vi "FLUKE_8845A.vi"() -> ()   [LabVIEW 2020]
uses:
  <vilib>/Instr/_visa.llb/VISA Configure Serial Port (Instr).vi
  <vilib>/Utility/file.llb/Write Delimited Spreadsheet (DBL).vi
panel:
  in  "Device 2":refnum<visa-resource-name>="COM4"
  in  "Function 2":u16(ring) caption="Function" items=["AC Current", "DC Current", "AC Voltage", "DC Voltage", "Resistance"]
  in  "Clear 2":bool
  in  "Save Stop 2":bool caption="Save Stop"
  in  "Save Start 2":bool caption="Save Start"
  out "Save Time 2":timestamp
  out "Save Data 2":dbl[](array[numeric]) caption="Save Data"
  out "Device2 Buffer":string
  out "Preview graph 2":cluster{dbl[], "array":dbl[]}(graph)
  out "Saving 2":bool caption="Saving"
  out "read buffer 2":string caption="Read Buffer"
  out "Change 2":bool caption="Change"
  in  "Save Path 2":path caption="Save Path"
  out "=> 2":bool
  out "OVERLOAD 2":bool caption="OVERLOAD"
  out "Preview graph":cluster{dbl[], "array":dbl[]}(graph)
  out "Save Time":timestamp
  in  "stop":bool
  out "OVERLOAD":bool
  out "=>":bool
  out "Device1 Buffer":string
  in  "Save Path":path
  in  "Clear":bool
  out "Change":bool
  out "Save Data":dbl[](array[numeric])
  out "Saving":bool
  in  "Save Stop":bool
  in  "Save Start":bool
  in  "Function":u16(ring) items=["AC Current", "DC Current", "AC Voltage", "DC Voltage", "Resistance"]
  out "read buffer":string caption="Read Buffer"
  in  "Device 1":refnum<visa-resource-name>="COM4"
  # "made by Ji Won Kim  2021.06.17"
  # "Digit Precision Multimeter Controller"
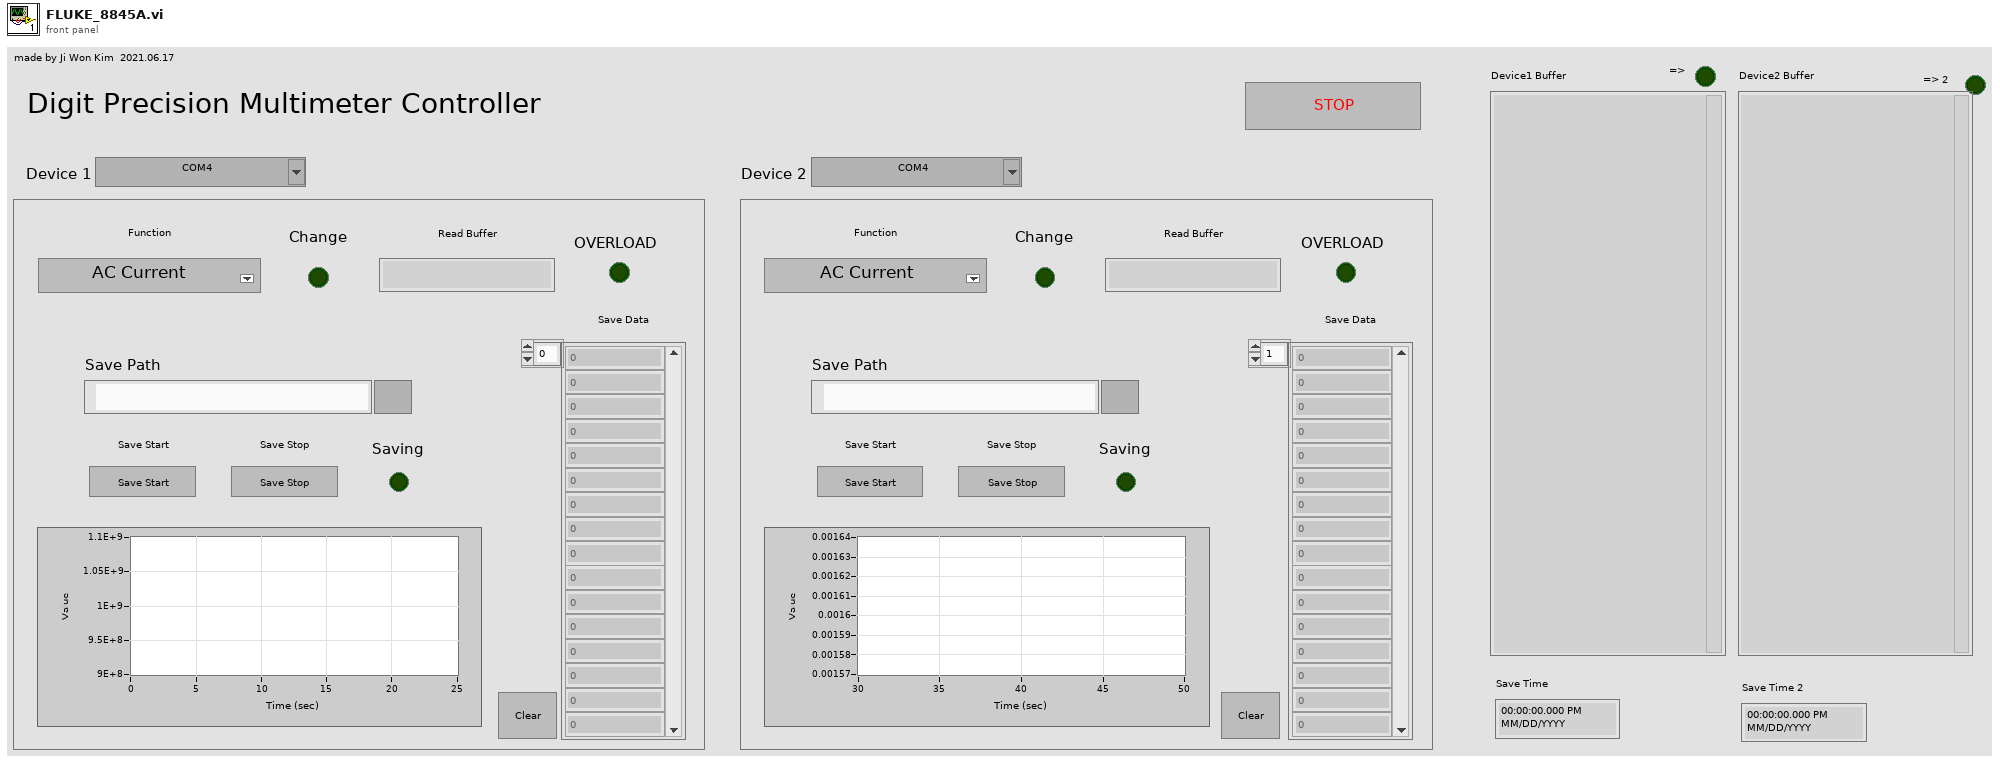
[diagram p1: front panel]
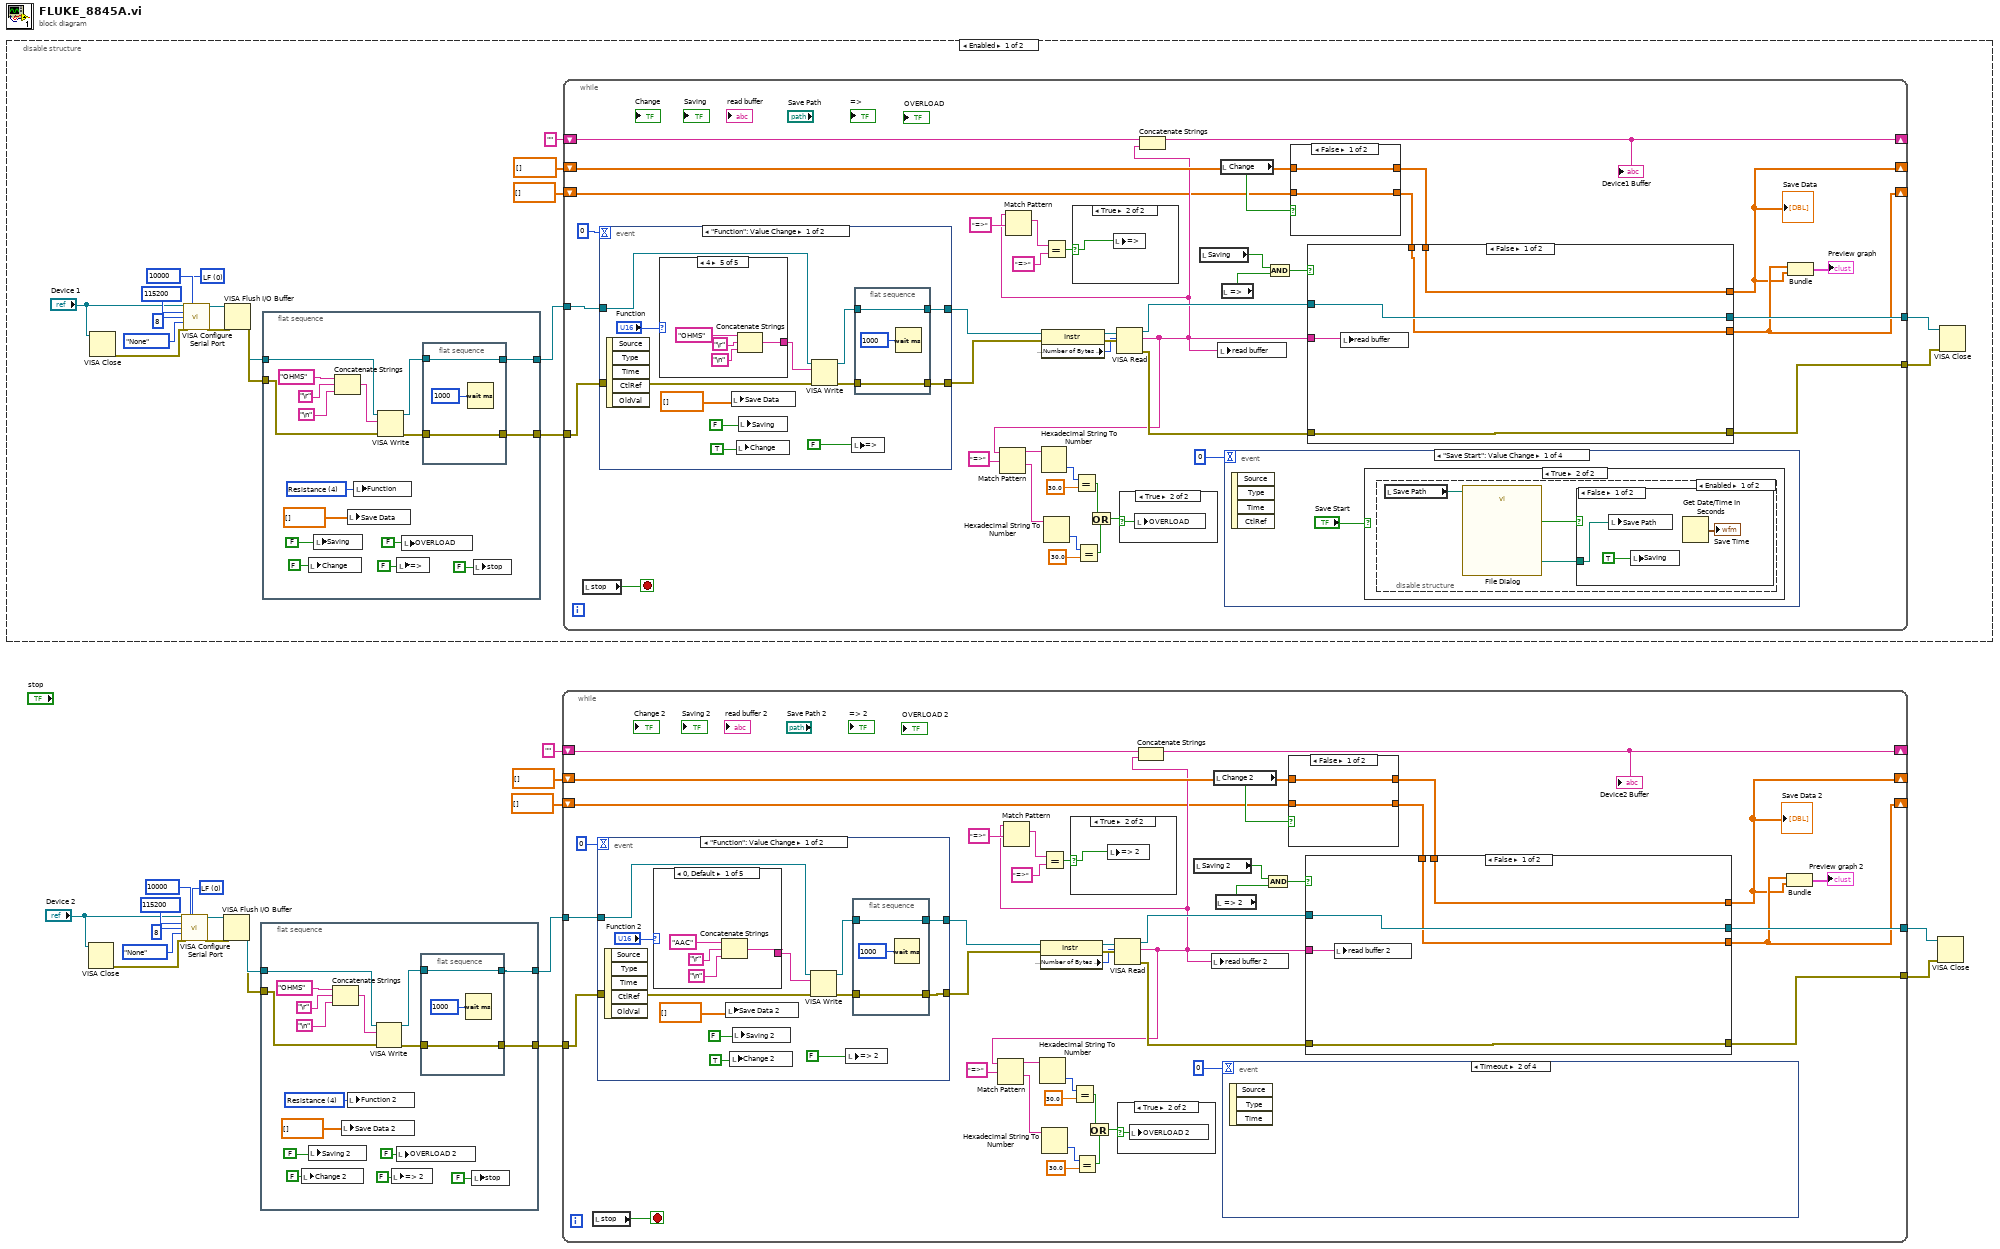
[diagram p0: block diagram]
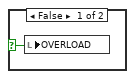
[diagram p2: hidden frame]
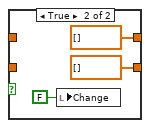
[diagram p4: hidden frame]
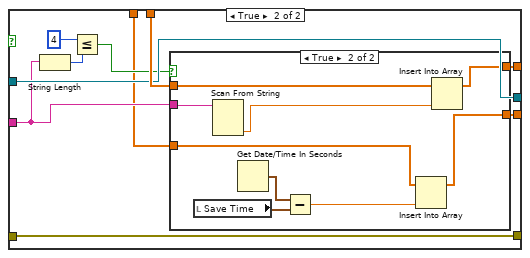
[diagram p5: hidden frame]
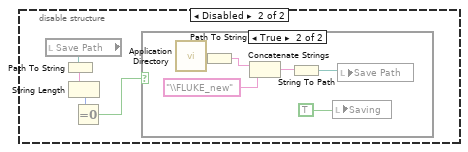
[diagram p9: hidden frame]
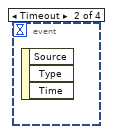
[diagram p11: hidden frame]
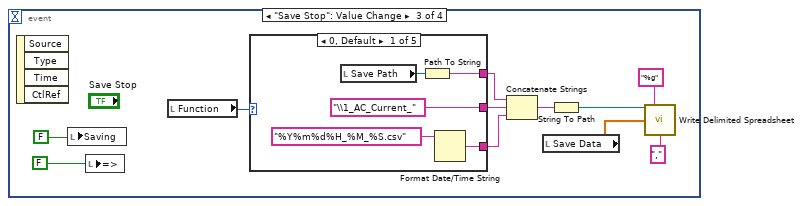
[diagram p12: hidden frame]
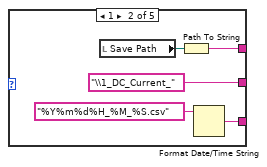
[diagram p13: hidden frame]
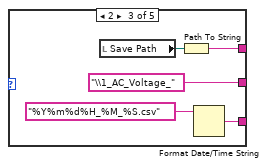
[diagram p14: hidden frame]
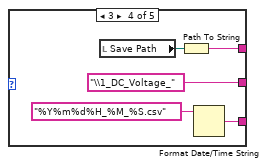
[diagram p15: hidden frame]
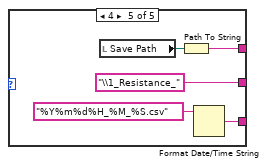
[diagram p16: hidden frame]
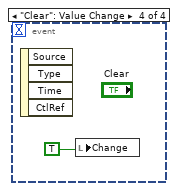
[diagram p17: hidden frame]
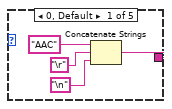
[diagram p18: hidden frame]
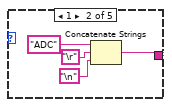
[diagram p19: hidden frame]
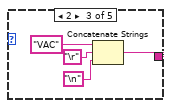
[diagram p20: hidden frame]
diagram:
  w3 = u16 0 items=["LF"]
  n1 = disable-structure shown="Enabled" {
    frame Enabled {
      w35 = u16 0 items=["LF"]
      n2 = VISA Close(VISA resource name="Device 1") -> (error out=w31:errorcluster)  [unwired: 1 in]
      n3 = call-poly "VISA Configure Serial Port"("VISA resource name"="Device 1", "timeout (10sec)"=u32 10000, "termination char\n(0xA = '\\n' = LF)"=w35, "baud rate (9600)"=u32 115200, "data bits (8)"=u16 8, "parity (0:none)"=enum16{"None", "Odd", "Even", "Mark", "Space"}."None", "error in (no error)"=w31) -> ("VISA resource name out"=w25:refnum<visa-resource-name>, "error out"=w24:errorcluster)  [unwired: 7 in]
      n4 = VISA Flush I/O Buffer(VISA resource name=w25, error in (no error)=w24) -> (VISA resource name out=w22:refnum<visa-resource-name>, error out=w23:errorcluster)  [unwired: 1 in]
      n5 = flat-sequence {
        tunnel: w22 -> [w46]
        tunnel: w23 -> [w45]
        tunnel: [w44] -> w27
        tunnel: [w43] -> w26
        frame #0 {
          w53 = u16 4 items=["AC Current", "DC Current", "AC Voltage", "DC Voltage", "Resistance"] ("Function")
          n6 = local write "Change"(FALSE ("Change")) -> ()
          n7 = local write "Saving"(FALSE ("Saving")) -> ()
          n8 = Concatenate Strings("OHMS" ("string"), "\r", "\n") -> (w52:string)
          n9 = local write "Save Data"(dbl[] [] ("array")) -> ()
          n10 = local write "Function"(w53) -> ()
          n11 = VISA Write(VISA resource name=w46, write buffer=w52, error in (no error)=w45) -> (VISA resource name out=w50:refnum<visa-resource-name>, error out=w51:errorcluster)  [unwired: 1 out]
          n12 = local write "=>"(FALSE ("Value Change")) -> ()
          n13 = local write "OVERLOAD"(FALSE ("OVERLOAD")) -> ()
          n14 = flat-sequence {
            tunnel: [w55] -> w44
            tunnel: w50 -> [w55]
            tunnel: [w54] -> w43
            tunnel: w51 -> [w54]
            frame #0 {
              n15 = Wait (ms)(milliseconds to wait=u32 1000) -> ()  [unwired: 1 out]
            }
          }
          n16 = local write "stop"(FALSE ("stop")) -> ()
        }
      }
      n17 = while {
        tunnel: [w88] -> w29
        tunnel: [w90] -> w28
        tunnel: w27 -> [w92]
        tunnel: w26 -> [w91]
        shift-right: [w57] -> _
        shift-left: dbl[] [] -> [w84]
        shift-right: [w82] -> _
        shift-left: "" -> [w81]
        shift-right: [w58] -> _
        shift-left: dbl[] [] ("array") -> [w60]
        stop <- w62 stop-if-true
        n18 = local read "stop"() -> (w62:bool)
        n19 = event shown="[0] \"Function\": Value Change" {
          selector: _ -> [_ _]
          dyn-events: _ -> [_ _]
          timeout: 0 -> [_ _]
          tunnel: [w196 w225] -> w95
          tunnel: [w194 w224] -> w94
          tunnel: w92 -> [w192 w223]
          tunnel: w91 -> [w191 w222]
          event "Function": Value Change {
            n20 = event-data() -> ()  [unwired: 1 in, 5 out]
            n21 = case shown="4" "Function" {
              tunnel: [w204 w208 w212 w216 w220] -> w197
              frame 0, Default {
                n22 = Concatenate Strings("AAC" ("string"), "\r", "\n") -> (w204:string)
              }
              frame 1 {
                n23 = Concatenate Strings("ADC" ("string"), "\r", "\n") -> (w208:string)
              }
              frame 2 {
                n24 = Concatenate Strings("VAC" ("string"), "\r", "\n") -> (w212:string)
              }
              frame 3 {
                n25 = Concatenate Strings("VDC" ("string"), "\r", "\n") -> (w216:string)
              }
              frame 4 {
                n26 = Concatenate Strings("OHMS" ("string"), "\r", "\n") -> (w220:string)
              }
            }
            n27 = local write "Save Data"(dbl[] [] ("array")) -> ()
            n28 = local write "Change"(TRUE ("Change")) -> ()
            n29 = local write "Saving"(FALSE ("Saving")) -> ()
            n30 = VISA Write(VISA resource name=w192, write buffer=w197, error in (no error)=w191) -> (VISA resource name out=w195:refnum<visa-resource-name>, error out=w193:errorcluster)  [unwired: 1 out]
            n31 = local write "=>"(FALSE ("Value Change")) -> ()
            n32 = flat-sequence {
              tunnel: [w199] -> w196
              tunnel: w195 -> [w199]
              tunnel: [w200] -> w194
              tunnel: w193 -> [w200]
              frame #0 {
                n33 = Wait (ms)(milliseconds to wait=u32 1000) -> ()  [unwired: 1 out]
              }
            }
          }
          event Timeout {
            n34 = event-data() -> ()  [unwired: 1 in, 3 out]
            n35 = Concatenate Strings("MEAS1?" ("string"), "\r", "\n") -> (w231:string)
            n36 = VISA Write(VISA resource name=w223, write buffer=w231, error in (no error)=w222) -> (VISA resource name out=w230:refnum<visa-resource-name>, error out=w229:errorcluster)  [unwired: 1 out]
            n37 = flat-sequence {
              tunnel: [w233] -> w225
              tunnel: w230 -> [w233]
              tunnel: [w232] -> w224
              tunnel: w229 -> [w232]
              frame #0 {
                n38 = Wait (ms)(milliseconds to wait=u32 1000) -> ()  [unwired: 1 out]
              }
            }
          }
        }
        n39 = property class="Instr"(reference=w95, error in=w94) -> (reference out=w98:refnum<visa-resource-name>, error out=w97:errorcluster, "Serial Settings:Number of Bytes at Serial Port"=w96:u32)
        n40 = VISA Read(VISA resource name=w98, byte count=w96, error in (no error)=w97) -> (VISA resource name out=w89:refnum<visa-resource-name>, read buffer=w73:string, error out=w87:errorcluster)  [unwired: 1 out]
        n41 = Match Pattern(string=w73, regular expression="=>" ("x")) -> (before substring=w69:string, after substring=w66:string)  [unwired: 1 in, 2 out]
        n42 = Match Pattern(string=w73, regular expression="=>" ("x")) -> (match substring=w77:string)  [unwired: 1 in, 3 out]
        n43 = Hexadecimal String To Number(string=w69) -> (number=w70:u32)  [unwired: 2 in, 1 out]
        n44 = Equal?(x=w77, y="=>" ("x")) -> (x = y?=w75:bool)
        n45 = Hexadecimal String To Number(string=w66) -> (number=w68:u32)  [unwired: 2 in, 1 out]
        n46 = case shown="True" w75 {
          selector: w75 -> [_ w101]
          frame False {
          }
          frame True {
            n47 = local write "=>"(w101) -> ()
          }
        }
        n48 = Equal?(x=w70, y=30.0) -> (x = y?=w65:bool)
        n49 = Equal?(x=w68, y=30.0) -> (x = y?=w64:bool)
        n50 = Or(x=w65, y=w64) -> (x .or. y?=w63:bool)
        n51 = case shown="True" w63 {
          selector: w63 -> [w99 w100]
          frame False {
            n52 = local write "OVERLOAD"(w99) -> ()
          }
          frame True {
            n53 = local write "OVERLOAD"(w100) -> ()
          }
        }
        n54 = Concatenate Strings(w81, w73) -> (w82:string)
        "Device1 Buffer" <- w82
        n55 = local read "Saving"() -> (w80:bool)
        n56 = local write "read buffer"(w73) -> ()
        n57 = local read "Change"() -> (w83:bool)
        n58 = local read "=>"() -> (w79:bool)
        n59 = event shown="[0] \"Save Start\": Value Change" {
          selector: _ -> [_ _ _ _]
          dyn-events: _ -> [_ _ _ _]
          timeout: 0 -> [_ _ _ _]
          event "Save Start": Value Change {
            n60 = event-data() -> ()  [unwired: 1 in, 4 out]
            n61 = case shown="True" "Save Start" {
              frame False {
              }
              frame True {
                n62 = disable-structure shown="Enabled" {
                  frame Enabled {
                    n63 = local read "Save Path"() -> (w134:path)
                    n64 = call "File Dialog"("start path"=w134) -> ("selected path"=w136:path, "cancelled"=w135:bool)  [unwired: 11 in, 2 out]
                    n65 = case shown="False" w135 {
                      tunnel: w136 -> [w138 _]
                      frame False {
                        n66 = local write "Save Path"(w138) -> ()
                        n67 = local write "Saving"(TRUE ("Saving")) -> ()
                        n68 = Get Date/Time In Seconds() -> (seconds since 1Jan1904=→"Save Time":timestamp)
                      }
                      frame True {
                      }
                    }
                  }
                  frame Disabled {
                    n69 = local read "Save Path"() -> (w143:path)
                    n70 = Path To String(path=w143) -> (string=w142:string)
                    n71 = String Length(string=w142) -> (length=w141:i32)
                    n72 = Equal To 0?(x=w141) -> (x = 0?=w140:bool)
                    n73 = case shown="True" w140 {
                      frame False {
                      }
                      frame True {
                        n74 = call <vilib>:"Application Directory.vi"() -> ("Application Directory"=w149:path)
                        n75 = Path To String(path=w149) -> (string=w148:string)
                        n76 = Concatenate Strings(w148, "\\FLUKE_new" ("string")) -> (w146:string)
                        n77 = String To Path(string=w146) -> (path=w145:path)
                        n78 = local write "Saving"(TRUE ("Saving")) -> ()
                        n79 = local write "Save Path"(w145) -> ()
                      }
                    }
                  }
                }
              }
            }
          }
          event Timeout {
            n80 = event-data() -> ()  [unwired: 1 in, 3 out]
          }
          event "Save Stop": Value Change {
            n81 = event-data() -> ()  [unwired: 1 in, 4 out]
            n82 = local write "Saving"(FALSE ("Saving")) -> ()
            n83 = local write "=>"(FALSE ("Value Change")) -> ()
            n84 = local read "Function"() -> (w155:u16)
            n85 = case shown="0, Default" w155 {
              tunnel: [w163 w168 w173 w178 w183] -> w156
              tunnel: ["\\1_AC_Current_" ("time format string (%c)") "\\1_DC_Current_" ("time format string (%c)") "\\1_AC_Voltage_" ("time format string (%c)") "\\1_DC_Voltage_" ("time format string (%c)") "\\1_Resistance_" ("time format string (%c)")] -> w157
              tunnel: [w161 w166 w171 w176 w181] -> w158
              frame 0, Default {
                n86 = local read "Save Path"() -> (w164:path)
                n87 = Path To String(path=w164) -> (string=w163:string)
                n88 = Format Date/Time String(time format string (%c)="%Y%m%d%H_%M_%S.csv") -> (date/time string=w161:string)  [unwired: 2 in]
              }
              frame 1 {
                n89 = local read "Save Path"() -> (w169:path)
                n90 = Path To String(path=w169) -> (string=w168:string)
                n91 = Format Date/Time String(time format string (%c)="%Y%m%d%H_%M_%S.csv") -> (date/time string=w166:string)  [unwired: 2 in]
              }
              frame 2 {
                n92 = local read "Save Path"() -> (w174:path)
                n93 = Path To String(path=w174) -> (string=w173:string)
                n94 = Format Date/Time String(time format string (%c)="%Y%m%d%H_%M_%S.csv") -> (date/time string=w171:string)  [unwired: 2 in]
              }
              frame 3 {
                n95 = local read "Save Path"() -> (w179:path)
                n96 = Path To String(path=w179) -> (string=w178:string)
                n97 = Format Date/Time String(time format string (%c)="%Y%m%d%H_%M_%S.csv") -> (date/time string=w176:string)  [unwired: 2 in]
              }
              frame 4 {
                n98 = local read "Save Path"() -> (w184:path)
                n99 = Path To String(path=w184) -> (string=w183:string)
                n100 = Format Date/Time String(time format string (%c)="%Y%m%d%H_%M_%S.csv") -> (date/time string=w181:string)  [unwired: 2 in]
              }
            }
            n101 = Concatenate Strings(w156, w157, w158) -> (w154:string)
            n102 = local read "Save Data"() -> (w151:dbl[])
            n103 = String To Path(string=w154) -> (path=w159:path)
            n104 = call-poly <vilib>:"Write Delimited Spreadsheet.vi"("file path (dialog if empty)"=w159, "format (%.3f)"="%g", "1D data"=w151, "delimiter (\\t)"="," ("delimiter (\\t)")) -> ()  [unwired: 10 in, 2 out]
          }
          event "Clear": Value Change {
            n105 = event-data() -> ()  [unwired: 1 in, 4 out]
            n106 = local write "Change"(TRUE ("Change")) -> ()
          }
        }
        n107 = And(x=w80, y=w79) -> (x .and. y?=w74:bool)
        n108 = case shown="False" w83 {
          tunnel: [w103 dbl[] []] -> w85
          tunnel: w84 -> [w103 _]
          tunnel: [w102 dbl[] [] ("array")] -> w61
          tunnel: w60 -> [w102 _]
          frame False {
          }
          frame True {
            n109 = local write "Change"(FALSE ("Change")) -> ()
          }
        }
        n110 = case shown="False" w74 {
          tunnel: w85 -> [w109 w121]
          tunnel: [w111 w120] -> w90
          tunnel: w89 -> [w111 w120]
          tunnel: [w110 w119] -> w88
          tunnel: w87 -> [w110 w119]
          tunnel: [w109 w118] -> w57
          tunnel: w73 -> [w108 w114]
          tunnel: w61 -> [w107 w113]
          tunnel: [w107 w112] -> w58
          frame False {
            n111 = local write "read buffer"(w108) -> ()
          }
          frame True {
            n112 = String Length(string=w114) -> (length=w117:i32)
            n113 = Less Or Equal?(x=4, y=w117) -> (x <= y?=w115:bool)
            n114 = case shown="True" w115 {
              tunnel: w121 -> [w123 w128]
              tunnel: [w123 w129] -> w118
              tunnel: w114 -> [_ w132]
              tunnel: w113 -> [w122 w125]
              tunnel: [w122 w124] -> w112
              frame False {
              }
              frame True {
                n115 = local read "Save Time"() -> (w130:timestamp)
                n116 = Scan From String(input string=w132) -> (output 1=w127:dbl)  [unwired: 4 in, 3 out]
                n117 = Get Date/Time In Seconds() -> (seconds since 1Jan1904=w131:timestamp)
                n118 = Subtract(x=w131, y=w130) -> (x-y=w126:dbl)
                n119 = Insert Into Array(array=w125, new element=w126) -> (w124:dbl[])  [unwired: 1 in]
                n120 = Insert Into Array(array=w128, new element=w127) -> (w129:dbl[])  [unwired: 1 in]
              }
            }
          }
        }
        "Save Data" <- w57
        n121 = Bundle("array"=w58, w57) -> (→"Preview graph":cluster{"array":dbl[], dbl[]})  [unwired: 1 in]
      }
      n122 = VISA Close(VISA resource name=w28, error in (no error)=w29) -> ()  [unwired: 1 out]
    }
    frame Disabled {
    }
  }
  n123 = VISA Close(VISA resource name="Device 2") -> (error out=w7:errorcluster)  [unwired: 1 in]
  n124 = call-poly "VISA Configure Serial Port"("VISA resource name"="Device 2", "timeout (10sec)"=u32 10000, "termination char\n(0xA = '\\n' = LF)"=w3, "baud rate (9600)"=u32 115200, "data bits (8)"=u16 8, "parity (0:none)"=enum16{"None", "Odd", "Even", "Mark", "Space"}."None", "error in (no error)"=w7) -> ("VISA resource name out"=w12:refnum<visa-resource-name>, "error out"=w13:errorcluster)  [unwired: 7 in]
  n125 = VISA Flush I/O Buffer(VISA resource name=w12, error in (no error)=w13) -> (VISA resource name out=w15:refnum<visa-resource-name>, error out=w14:errorcluster)  [unwired: 1 in]
  n126 = flat-sequence {
    tunnel: w15 -> [w244]
    tunnel: w14 -> [w243]
    tunnel: [w242] -> w10
    tunnel: [w241] -> w11
    frame #0 {
      w251 = u16 4 items=["AC Current", "DC Current", "AC Voltage", "DC Voltage", "Resistance"] ("Function")
      n127 = local write "Change 2"(FALSE ("Change")) -> ()
      n128 = local write "Saving 2"(FALSE ("Saving")) -> ()
      n129 = Concatenate Strings("OHMS" ("string"), "\r", "\n") -> (w250:string)
      n130 = local write "Save Data 2"(dbl[] [] ("array")) -> ()
      n131 = local write "Function 2"(w251) -> ()
      n132 = VISA Write(VISA resource name=w244, write buffer=w250, error in (no error)=w243) -> (VISA resource name out=w248:refnum<visa-resource-name>, error out=w249:errorcluster)  [unwired: 1 out]
      n133 = local write "=> 2"(FALSE ("Value Change")) -> ()
      n134 = local write "OVERLOAD 2"(FALSE ("OVERLOAD")) -> ()
      n135 = flat-sequence {
        tunnel: [w253] -> w242
        tunnel: w248 -> [w253]
        tunnel: [w252] -> w241
        tunnel: w249 -> [w252]
        frame #0 {
          n136 = Wait (ms)(milliseconds to wait=u32 1000) -> ()  [unwired: 1 out]
        }
      }
      n137 = local write "stop"(FALSE ("stop")) -> ()
    }
  }
  n138 = while {
    tunnel: [w286] -> w8
    tunnel: [w288] -> w9
    tunnel: w10 -> [w290]
    tunnel: w11 -> [w289]
    shift-right: [w255] -> _
    shift-left: dbl[] [] -> [w282]
    shift-right: [w280] -> _
    shift-left: "" -> [w279]
    shift-right: [w256] -> _
    shift-left: dbl[] [] ("array") -> [w258]
    stop <- w260 stop-if-true
    n139 = local read "stop"() -> (w260:bool)
    n140 = event shown="[0] \"Function\": Value Change" {
      selector: _ -> [_ _]
      dyn-events: _ -> [_ _]
      timeout: 0 -> [_ _]
      tunnel: [w394 w423] -> w293
      tunnel: [w392 w422] -> w292
      tunnel: w290 -> [w390 w421]
      tunnel: w289 -> [w389 w420]
      event "Function": Value Change {
        n141 = event-data() -> ()  [unwired: 1 in, 5 out]
        n142 = case shown="0, Default" "Function 2" {
          tunnel: [w402 w406 w410 w414 w418] -> w395
          frame 0, Default {
            n143 = Concatenate Strings("AAC" ("string"), "\r", "\n") -> (w402:string)
          }
          frame 1 {
            n144 = Concatenate Strings("ADC" ("string"), "\r", "\n") -> (w406:string)
          }
          frame 2 {
            n145 = Concatenate Strings("VAC" ("string"), "\r", "\n") -> (w410:string)
          }
          frame 3 {
            n146 = Concatenate Strings("VDC" ("string"), "\r", "\n") -> (w414:string)
          }
          frame 4 {
            n147 = Concatenate Strings("OHMS" ("string"), "\r", "\n") -> (w418:string)
          }
        }
        n148 = local write "Save Data 2"(dbl[] [] ("array")) -> ()
        n149 = local write "Change 2"(TRUE ("Change")) -> ()
        n150 = local write "Saving 2"(FALSE ("Saving")) -> ()
        n151 = VISA Write(VISA resource name=w390, write buffer=w395, error in (no error)=w389) -> (VISA resource name out=w393:refnum<visa-resource-name>, error out=w391:errorcluster)  [unwired: 1 out]
        n152 = local write "=> 2"(FALSE ("Value Change")) -> ()
        n153 = flat-sequence {
          tunnel: [w397] -> w394
          tunnel: w393 -> [w397]
          tunnel: [w398] -> w392
          tunnel: w391 -> [w398]
          frame #0 {
            n154 = Wait (ms)(milliseconds to wait=u32 1000) -> ()  [unwired: 1 out]
          }
        }
      }
      event Timeout {
        n155 = event-data() -> ()  [unwired: 1 in, 3 out]
        n156 = Concatenate Strings("MEAS1?" ("string"), "\r", "\n") -> (w429:string)
        n157 = VISA Write(VISA resource name=w421, write buffer=w429, error in (no error)=w420) -> (VISA resource name out=w428:refnum<visa-resource-name>, error out=w427:errorcluster)  [unwired: 1 out]
        n158 = flat-sequence {
          tunnel: [w431] -> w423
          tunnel: w428 -> [w431]
          tunnel: [w430] -> w422
          tunnel: w427 -> [w430]
          frame #0 {
            n159 = Wait (ms)(milliseconds to wait=u32 1000) -> ()  [unwired: 1 out]
          }
        }
      }
    }
    n160 = property class="Instr"(reference=w293, error in=w292) -> (reference out=w296:refnum<visa-resource-name>, error out=w295:errorcluster, "Serial Settings:Number of Bytes at Serial Port"=w294:u32)
    n161 = VISA Read(VISA resource name=w296, byte count=w294, error in (no error)=w295) -> (VISA resource name out=w287:refnum<visa-resource-name>, read buffer=w271:string, error out=w285:errorcluster)  [unwired: 1 out]
    n162 = Match Pattern(string=w271, regular expression="=>" ("x")) -> (before substring=w267:string, after substring=w264:string)  [unwired: 1 in, 2 out]
    n163 = Match Pattern(string=w271, regular expression="=>" ("x")) -> (match substring=w275:string)  [unwired: 1 in, 3 out]
    n164 = Hexadecimal String To Number(string=w267) -> (number=w268:u32)  [unwired: 2 in, 1 out]
    n165 = Equal?(x=w275, y="=>" ("x")) -> (x = y?=w273:bool)
    n166 = Hexadecimal String To Number(string=w264) -> (number=w266:u32)  [unwired: 2 in, 1 out]
    n167 = case shown="True" w273 {
      selector: w273 -> [_ w299]
      frame False {
      }
      frame True {
        n168 = local write "=> 2"(w299) -> ()
      }
    }
    n169 = Equal?(x=w268, y=30.0) -> (x = y?=w263:bool)
    n170 = Equal?(x=w266, y=30.0) -> (x = y?=w262:bool)
    n171 = Or(x=w263, y=w262) -> (x .or. y?=w261:bool)
    n172 = case shown="True" w261 {
      selector: w261 -> [w297 w298]
      frame False {
        n173 = local write "OVERLOAD 2"(w297) -> ()
      }
      frame True {
        n174 = local write "OVERLOAD 2"(w298) -> ()
      }
    }
    n175 = Concatenate Strings(w279, w271) -> (w280:string)
    "Device2 Buffer" <- w280
    n176 = local read "Saving 2"() -> (w278:bool)
    n177 = local write "read buffer 2"(w271) -> ()
    n178 = local read "Change 2"() -> (w281:bool)
    n179 = local read "=> 2"() -> (w277:bool)
    n180 = event shown="[1] Timeout" {
      selector: _ -> [_ _ _ _]
      dyn-events: _ -> [_ _ _ _]
      timeout: 0 -> [_ _ _ _]
      event "Save Start": Value Change {
        n181 = event-data() -> ()  [unwired: 1 in, 4 out]
        n182 = case shown="True" "Save Start 2" {
          frame False {
          }
          frame True {
            n183 = disable-structure shown="Enabled" {
              frame Enabled {
                n184 = local read "Save Path 2"() -> (w332:path)
                n185 = call "File Dialog2"("start path"=w332) -> ("selected path"=w334:path, "cancelled"=w333:bool)  [unwired: 11 in, 2 out]
                n186 = case shown="False" w333 {
                  tunnel: w334 -> [w336 _]
                  frame False {
                    n187 = local write "Save Path 2"(w336) -> ()
                    n188 = local write "Saving 2"(TRUE ("Saving")) -> ()
                    n189 = Get Date/Time In Seconds() -> (seconds since 1Jan1904=→"Save Time 2":timestamp)
                  }
                  frame True {
                  }
                }
              }
              frame Disabled {
                n190 = local read "Save Path 2"() -> (w341:path)
                n191 = Path To String(path=w341) -> (string=w340:string)
                n192 = String Length(string=w340) -> (length=w339:i32)
                n193 = Equal To 0?(x=w339) -> (x = 0?=w338:bool)
                n194 = case shown="True" w338 {
                  frame False {
                  }
                  frame True {
                    n195 = call <vilib>:"Application Directory.vi"() -> ("Application Directory"=w347:path)
                    n196 = Path To String(path=w347) -> (string=w346:string)
                    n197 = Concatenate Strings(w346, "\\FLUKE_new" ("string")) -> (w344:string)
                    n198 = String To Path(string=w344) -> (path=w343:path)
                    n199 = local write "Saving 2"(TRUE ("Saving")) -> ()
                    n200 = local write "Save Path 2"(w343) -> ()
                  }
                }
              }
            }
          }
        }
      }
      event Timeout {
        n201 = event-data() -> ()  [unwired: 1 in, 3 out]
      }
      event "Save Stop": Value Change {
        n202 = event-data() -> ()  [unwired: 1 in, 4 out]
        n203 = local write "Saving 2"(FALSE ("Saving")) -> ()
        n204 = local write "=> 2"(FALSE ("Value Change")) -> ()
        n205 = local read "Function 2"() -> (w353:u16)
        n206 = case shown="3" w353 {
          tunnel: [w361 w366 w371 w376 w381] -> w354
          tunnel: ["\\2_AC_Current_" ("time format string (%c)") "\\2_DC_Current_" ("time format string (%c)") "\\2_AC_Voltage_" ("time format string (%c)") "\\2_DC_Voltage_" ("time format string (%c)") "\\2_Resistance_" ("time format string (%c)")] -> w355
          tunnel: [w359 w364 w369 w374 w379] -> w356
          frame 0, Default {
            n207 = local read "Save Path 2"() -> (w362:path)
            n208 = Path To String(path=w362) -> (string=w361:string)
            n209 = Format Date/Time String(time format string (%c)="%Y%m%d%H_%M_%S.csv") -> (date/time string=w359:string)  [unwired: 2 in]
          }
          frame 1 {
            n210 = local read "Save Path 2"() -> (w367:path)
            n211 = Path To String(path=w367) -> (string=w366:string)
            n212 = Format Date/Time String(time format string (%c)="%Y%m%d%H_%M_%S.csv") -> (date/time string=w364:string)  [unwired: 2 in]
          }
          frame 2 {
            n213 = local read "Save Path 2"() -> (w372:path)
            n214 = Path To String(path=w372) -> (string=w371:string)
            n215 = Format Date/Time String(time format string (%c)="%Y%m%d%H_%M_%S.csv") -> (date/time string=w369:string)  [unwired: 2 in]
          }
          frame 3 {
            n216 = local read "Save Path 2"() -> (w377:path)
            n217 = Path To String(path=w377) -> (string=w376:string)
            n218 = Format Date/Time String(time format string (%c)="%Y%m%d%H_%M_%S.csv") -> (date/time string=w374:string)  [unwired: 2 in]
          }
          frame 4 {
            n219 = local read "Save Path 2"() -> (w382:path)
            n220 = Path To String(path=w382) -> (string=w381:string)
            n221 = Format Date/Time String(time format string (%c)="%Y%m%d%H_%M_%S.csv") -> (date/time string=w379:string)  [unwired: 2 in]
          }
        }
        n222 = Concatenate Strings(w354, w355, w356) -> (w352:string)
        n223 = local read "Save Data 2"() -> (w349:dbl[])
        n224 = String To Path(string=w352) -> (path=w357:path)
        n225 = call-poly <vilib>:"Write Delimited Spreadsheet.vi"("file path (dialog if empty)"=w357, "format (%.3f)"="%g", "1D data"=w349, "delimiter (\\t)"="," ("delimiter (\\t)")) -> ()  [unwired: 10 in, 2 out]
      }
      event "Clear": Value Change {
        n226 = event-data() -> ()  [unwired: 1 in, 4 out]
        n227 = local write "Change 2"(TRUE ("Change")) -> ()
      }
    }
    n228 = And(x=w278, y=w277) -> (x .and. y?=w272:bool)
    n229 = case shown="False" w281 {
      tunnel: [w301 dbl[] []] -> w283
      tunnel: w282 -> [w301 _]
      tunnel: [w300 dbl[] [] ("array")] -> w259
      tunnel: w258 -> [w300 _]
      frame False {
      }
      frame True {
        n230 = local write "Change 2"(FALSE ("Change")) -> ()
      }
    }
    n231 = case shown="False" w272 {
      tunnel: w283 -> [w307 w319]
      tunnel: [w309 w318] -> w288
      tunnel: w287 -> [w309 w318]
      tunnel: [w308 w317] -> w286
      tunnel: w285 -> [w308 w317]
      tunnel: [w307 w316] -> w255
      tunnel: w271 -> [w306 w312]
      tunnel: w259 -> [w305 w311]
      tunnel: [w305 w310] -> w256
      frame False {
        n232 = local write "read buffer 2"(w306) -> ()
      }
      frame True {
        n233 = String Length(string=w312) -> (length=w315:i32)
        n234 = Less Or Equal?(x=4, y=w315) -> (x <= y?=w313:bool)
        n235 = case shown="True" w313 {
          tunnel: w319 -> [w321 w326]
          tunnel: [w321 w327] -> w316
          tunnel: w312 -> [_ w330]
          tunnel: w311 -> [w320 w323]
          tunnel: [w320 w322] -> w310
          frame False {
          }
          frame True {
            n236 = local read "Save Time 2"() -> (w328:timestamp)
            n237 = Scan From String(input string=w330) -> (output 1=w325:dbl)  [unwired: 4 in, 3 out]
            n238 = Get Date/Time In Seconds() -> (seconds since 1Jan1904=w329:timestamp)
            n239 = Subtract(x=w329, y=w328) -> (x-y=w324:dbl)
            n240 = Insert Into Array(array=w323, new element=w324) -> (w322:dbl[])  [unwired: 1 in]
            n241 = Insert Into Array(array=w326, new element=w325) -> (w327:dbl[])  [unwired: 1 in]
          }
        }
      }
    }
    "Save Data 2" <- w255
    n242 = Bundle("array"=w256, w255) -> (→"Preview graph 2":cluster{"array":dbl[], dbl[]})  [unwired: 1 in]
  }
  n243 = VISA Close(VISA resource name=w9, error in (no error)=w8) -> ()  [unwired: 1 out]
